vi "Main.vi"() -> ()   [LabVIEW 2019]
doc: "Use this template to build a simple state machine design pattern. Each state executes code and determines which state to transition to."
uses:
  controls/Data.ctl
  controls/State.ctl
  <vilib>/Utility/miscctls.llb/LVPointTypeDef.ctl
panel:
  in  "Prompt Empty":bool
  in  "History":bool
  in  "Advanced":bool
  out "NextEffect3":picture
  out "NextEffect2":picture
  out "NextEffect1":picture
  out "Effect3":picture
  out "Effect2":picture
  out "Effect1":picture
  out "Title":picture
  out "Player Aid":picture
  out "Discard":i32 caption="Discard Deck Size"
  out "Draw":i32 caption="Draw Deck Size"
  out "Value 3":i32
  out "Value 2":i32
  out "Value 1":i32
  in  "Player Reshuffle":bool
  out "Error":errorcluster
  in  "Exit":bool
  in  "Draw Next":bool
  in  "Reset":bool
  out "Scoring3":picture
  out "Scoring2":picture
  out "Scoring1":picture
  out "NumberBack3":picture
  out "NumberBack2":picture
  out "NumberBack1":picture
  out "EffectBack3":picture
  out "EffectBack2":picture
  out "EffectBack1":picture
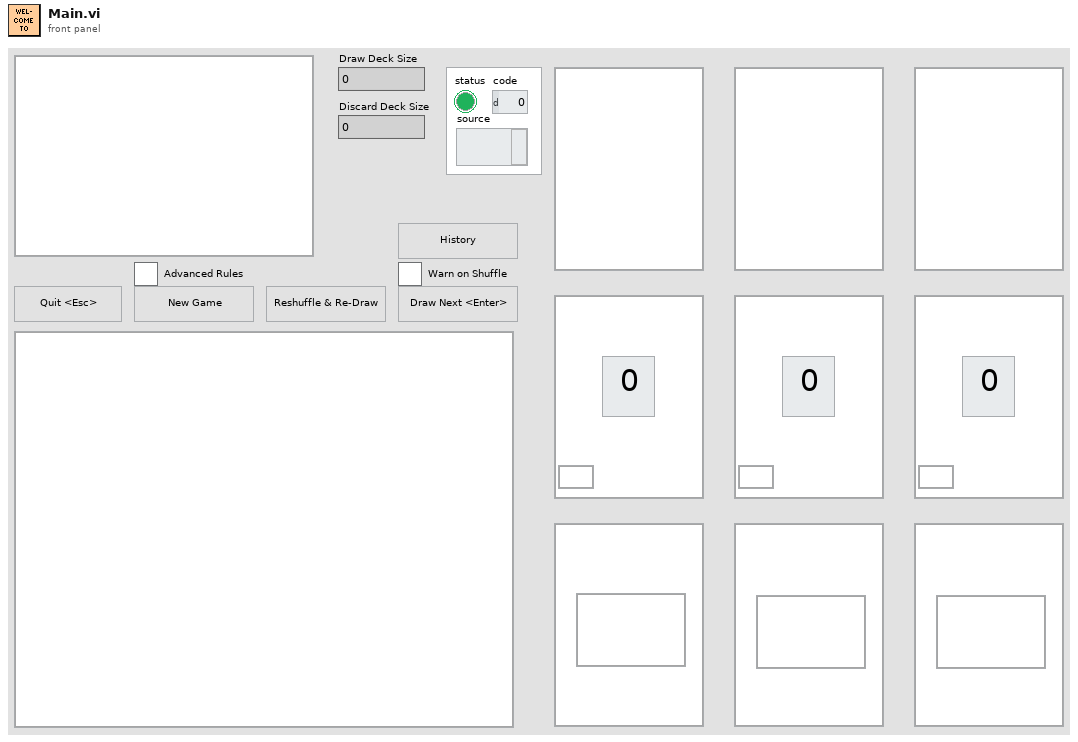
[diagram p1: front panel]
types:
  T1 = typedef "State.ctl" = enum16{"Initialize", "Draw Next Cards", "Shuffle", "Update Display", "Wait for Event", "Reset", "Error", "Exit"}
  T2 = typedef "Data.ctl" = cluster{"Draw Deck":variant[], "Discard Deck":variant[], "Effect Images":variant, "Cards In Draw Deck":i32, "City Card Deck":variant[]}
  T3 = typedef "LVPointTypeDef.ctl" = cluster{"Horizontal":i16, "Vertical":i16}
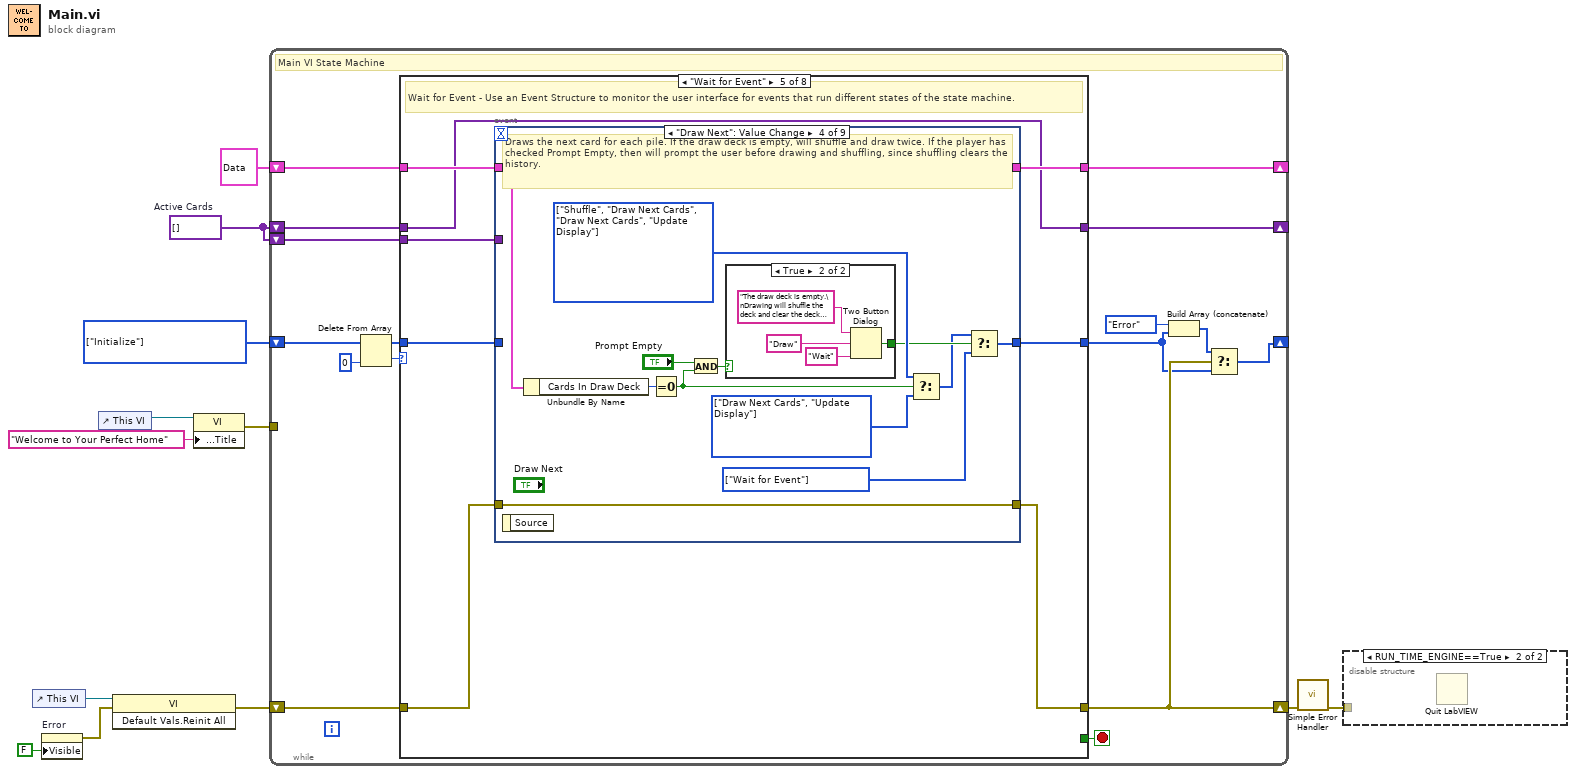
[diagram p0: block diagram]
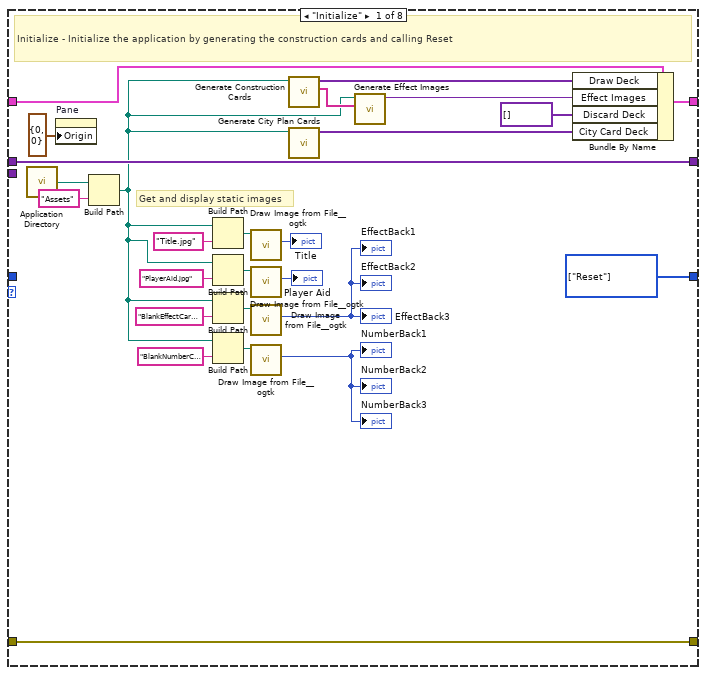
[diagram p3: hidden frame]
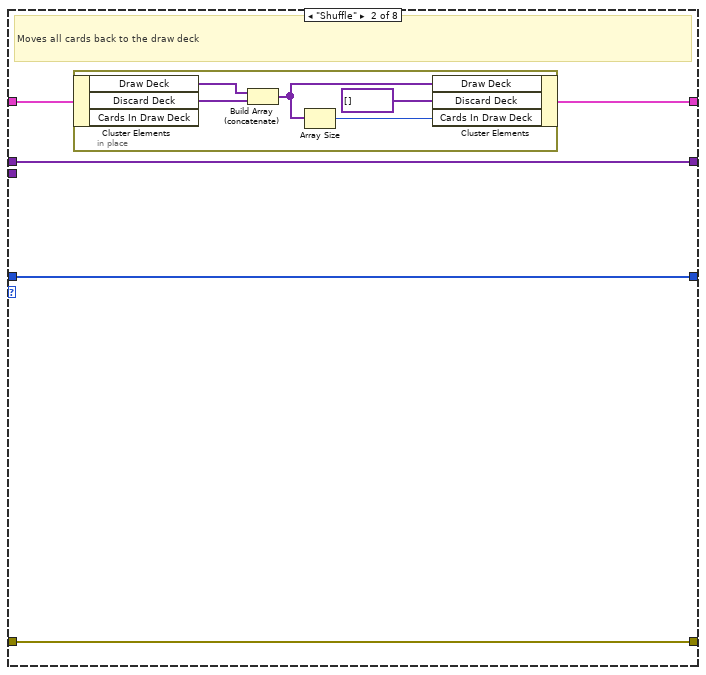
[diagram p4: hidden frame]
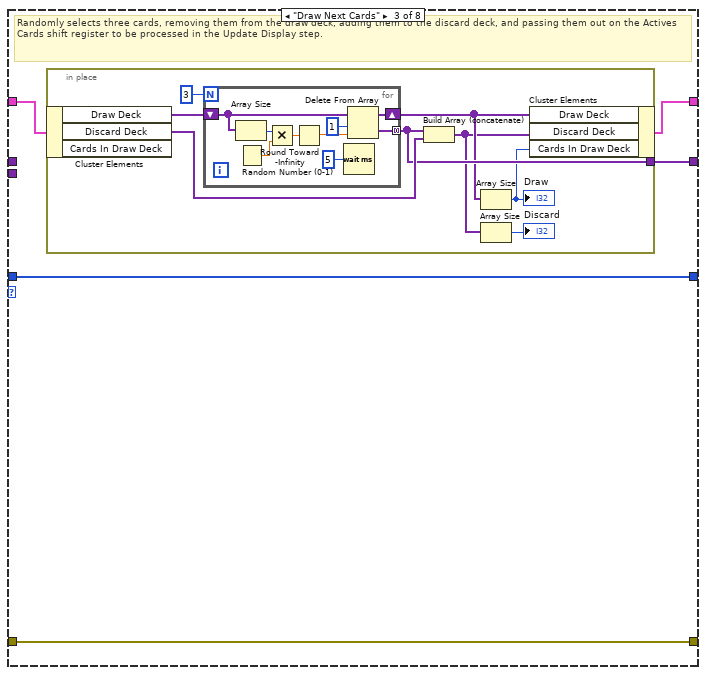
[diagram p5: hidden frame]
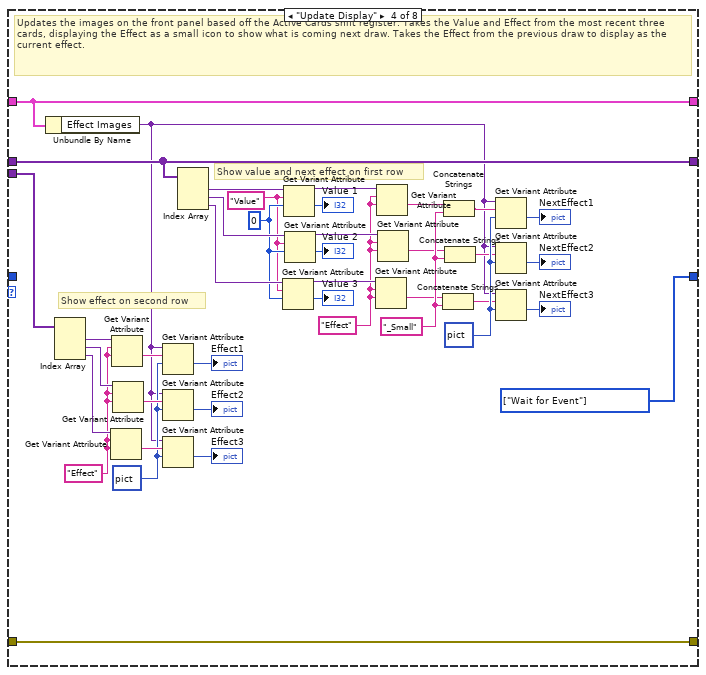
[diagram p6: hidden frame]
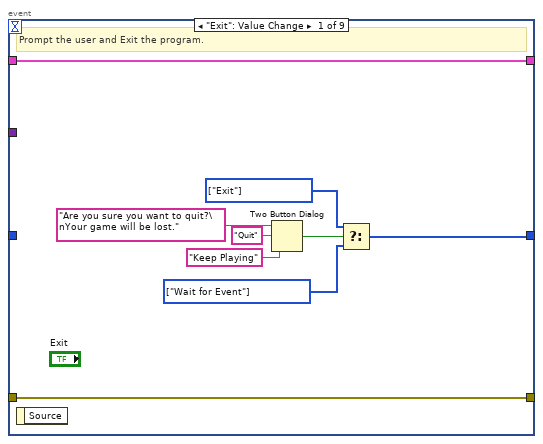
[diagram p7: hidden frame]
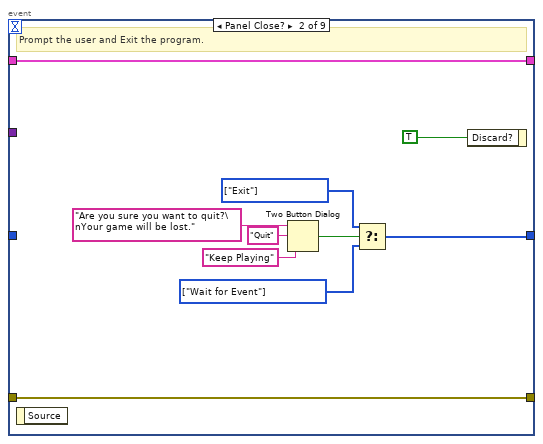
[diagram p8: hidden frame]
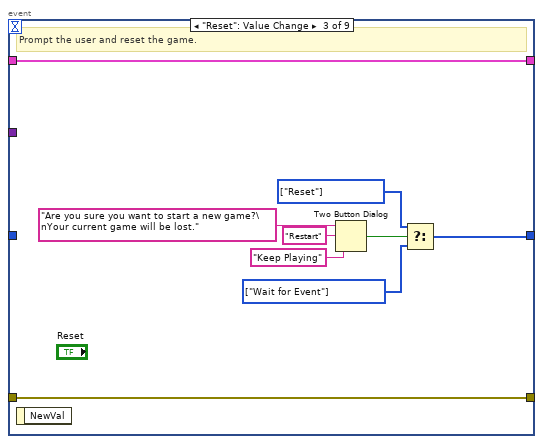
[diagram p9: hidden frame]
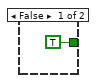
[diagram p10: hidden frame]
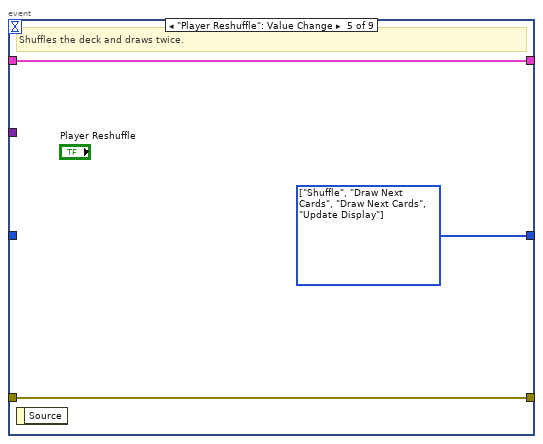
[diagram p11: hidden frame]
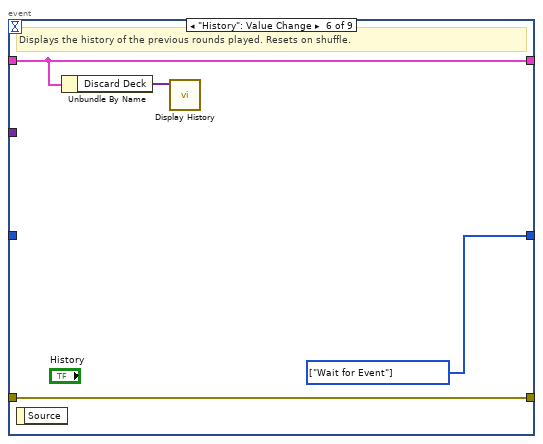
[diagram p12: hidden frame]
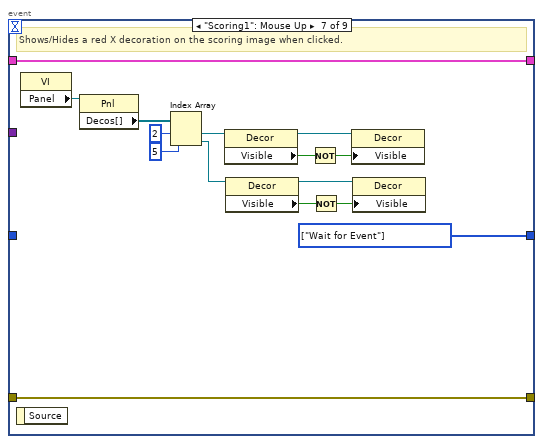
[diagram p13: hidden frame]
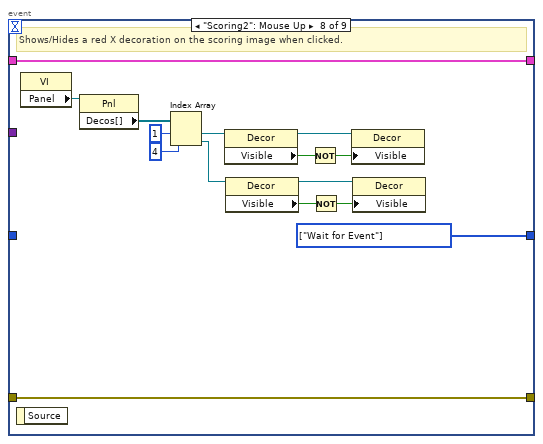
[diagram p14: hidden frame]
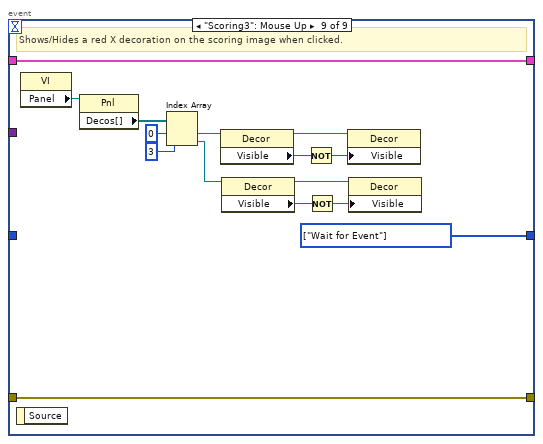
[diagram p15: hidden frame]
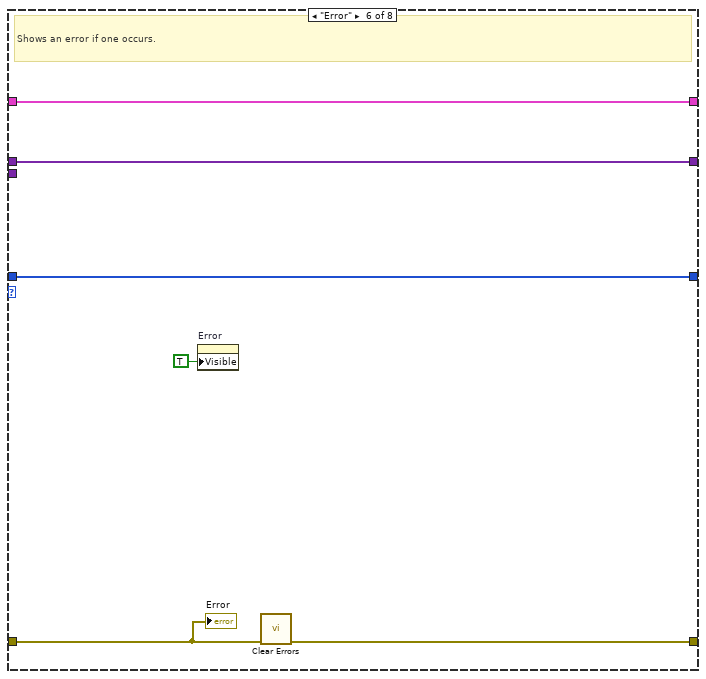
[diagram p16: hidden frame]
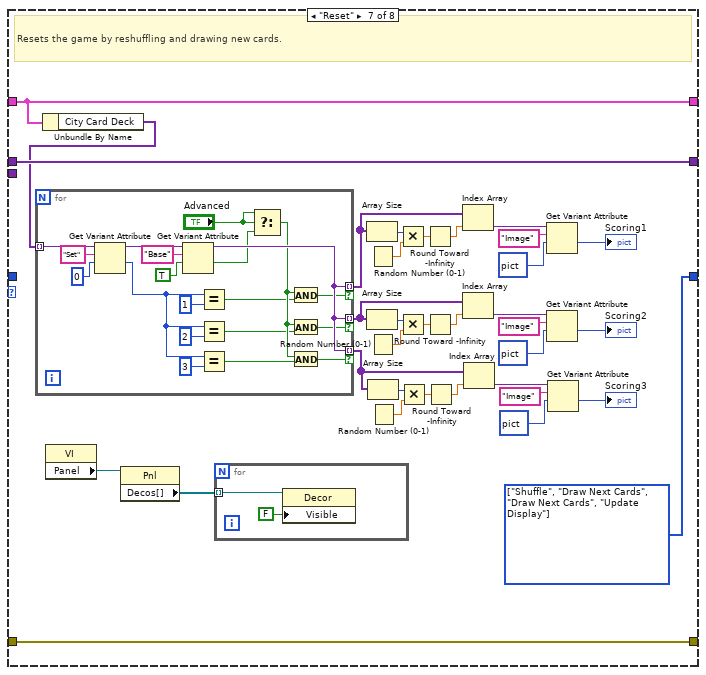
[diagram p17: hidden frame]
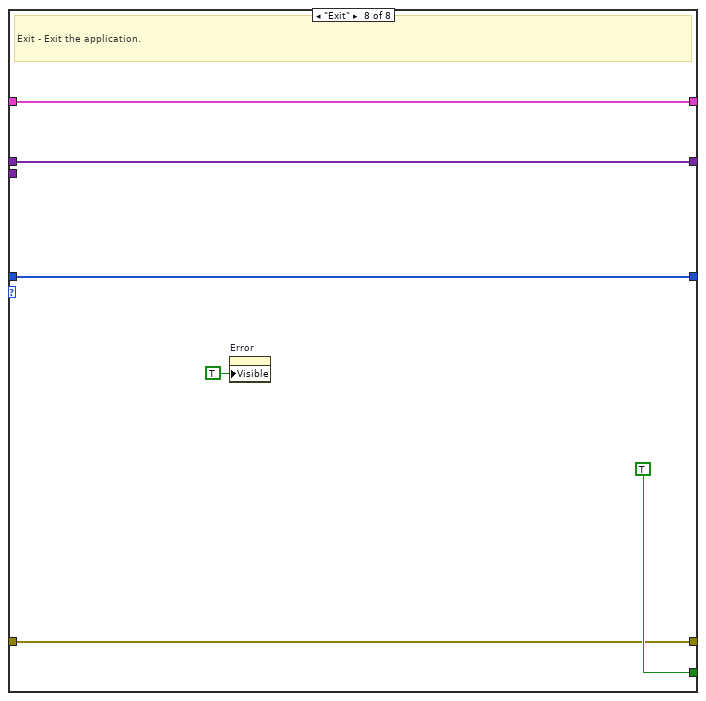
[diagram p18: hidden frame]
diagram:
  w4 = variant[] []  # Active Cards
  w9 = T1[] [enum."Initialize"] items=["Initialize", "Draw Next Cards", "Shuffle", "Update Display", "Wait for Event", "Reset", "Error", "Exit"]
  n1 = control-ref of="This VI"() -> (w8:refnum<vi>)
  n2 = property on="Error" class="Clust (strict)"("Visible"=FALSE) -> (error out=w5:errorcluster)  [unwired: 2 in, 1 out]
  n3 = control-ref of="This VI"() -> (w3:refnum<vi>)
  n4 = invoke class="VI" method="Default Vals.Reinit All"(reference=w8, error in=w5) -> (error out=w7:errorcluster)  [unwired: 1 in, 2 out]
  n5 = property class="VI"(reference=w3, "Front Panel.Title"="Welcome to Your Perfect Home" ("Front Panel Window:Title")) -> (error out=w1:errorcluster)  [unwired: 1 in, 1 out]
  n6 = while {
    shift-right: [w18] -> _
    shift-left: w9 -> [w23]
    shift-right: [w27] -> _
    shift-left: T2 {"Draw Deck"=[], "Discard Deck"=[], "Effect Images"=variant(variant[] []), "Cards In Draw Deck"=0, "City Card Deck"=[]} ("Data") -> [w28]
    shift-right: [w24] -> w11
    shift-left: w7 -> [w26]
    shift-right: [w15] -> _
    shift-left: w4 -> [w14]
    shift-left: w4 -> [w13]
    tunnel: w1 -> [_]
    stop <- w25 stop-if-true
    # "Main VI State Machine"
    n7 = Delete From Array(array=w23, index=0) -> (deleted portion=w21:T1, array with subset deleted=w20:T1[])  [unwired: 1 in]
    n8 = case shown="\"Wait for Event\"" w21 {
      tunnel: [w53 w58 w65 w125 w134 w236 w270 w296] -> w16
      tunnel: [_ _ _ _ _ _ _ TRUE ("Stop Loop")] -> w25
      tunnel: w28 -> [w33 w57 w68 w110 w133 w237 w268 w299]
      tunnel: [w52 w56 w67 w110 w132 w237 w268 w299] -> w27
      tunnel: w26 -> [w54 w59 w69 w126 w131 w234 w271 w297]
      tunnel: [w54 w59 w69 w126 w130 w233 w271 w297] -> w24
      tunnel: w20 -> [_ w58 w65 _ w129 w236 _ w296]
      tunnel: [w51 w55 w66 w121 w128 w232 w269 w294] -> w15
      tunnel: w14 -> [w51 w55 _ w121 w128 w232 w269 w294]
      tunnel: w13 -> [_ _ _ w114 w127 _ _ _]
      frame "Initialize" {
        w53 = T1[] [enum."Reset"] items=["Initialize", "Draw Next Cards", "Shuffle", "Update Display", "Wait for Event", "Reset", "Error", "Exit"] ("Array")
        # "Get and display static images"
        # "Initialize - Initialize the application by generating the construction cards and calling Reset"
        n9 = call <vilib>:"Application Directory.vi"() -> ("Application Directory"=w50:path)
        n10 = property on="Pane" class="Pane"("Origin"=T3 {"Horizontal"=0, "Vertical"=0}) -> ()  [unwired: 2 in, 2 out]
        n11 = Build Path(base path=w50, name or relative path="Assets") -> (appended path=w29:path)
        n12 = Build Path(base path=w29, name or relative path="Title.jpg") -> (appended path=w47:path)
        n13 = Build Path(base path=w29, name or relative path="PlayerAid.jpg") -> (appended path=w45:path)
        n14 = Build Path(base path=w29, name or relative path="BlankEffectCard.jpg") -> (appended path=w40:path)
        n15 = Build Path(base path=w29, name or relative path="BlankNumberCard.jpg") -> (appended path=w39:path)
        n16 = call <userlib>:"Draw Image from File__ogtk.vi"("path to image file"=w47) -> ("new picture"=→"Title":picture)  [unwired: 7 in, 3 out]
        n17 = call <userlib>:"Draw Image from File__ogtk.vi"("path to image file"=w45) -> ("new picture"=→"Player Aid":picture)  [unwired: 7 in, 3 out]
        n18 = call <userlib>:"Draw Image from File__ogtk.vi"("path to image file"=w40) -> ("new picture"=→"EffectBack2" →"EffectBack3" →"EffectBack1":picture)  [unwired: 7 in, 3 out]
        n19 = call <userlib>:"Draw Image from File__ogtk.vi"("path to image file"=w39) -> ("new picture"=→"NumberBack2" →"NumberBack3" →"NumberBack1":picture)  [unwired: 7 in, 3 out]
        n20 = call "Generate Construction Cards.vi"("Path"=w29) -> ("Effect Types"=w35:string[], "Construction Cards"=w32:variant[])  [unwired: 9 in]
        n21 = call "Generate City Plan Cards.vi"("Path"=w29) -> ("City Plan Cards"=w34:variant[])  [unwired: 10 in]
        n22 = call "Generate Effect Images.vi"("Effect Types"=w35, "Path"=w29) -> ("Effect Images"=w31:variant)  [unwired: 9 in]
        n23 = Bundle By Name(cluster=w33, "Draw Deck"=w32, "Effect Images"=w31, "Discard Deck"=variant[] [], "City Card Deck"=w34) -> (w52:T2)
      }
      frame "Shuffle" {
        # "Moves all cards back to the draw deck"
        n24 = in-place {
          n25 = in-place-cluster #1(w57) -> ("Draw Deck"=w62:variant[], "Discard Deck"=w63:variant[])  [unwired: 1 out]
          n26 = Build Array (concatenate)(w62, w63) -> (w60:variant[])
          n27 = Array Size(array=w60) -> (size(s)=w61:i32)
          n28 = in-place-cluster #1("Draw Deck"=w60, "Discard Deck"=variant[] [], "Cards In Draw Deck"=w61) -> (w56:T2)
        }
      }
      frame "Draw Next Cards" {
        # "Randomly selects three cards, removing them from the draw deck, adding them to the discard deck, and passing them out on the Actives Cards shift register to be processed in the Update Display step."
        n29 = in-place {
          in-place-border: [w74] -> w66
          n30 = in-place-cluster #2(w68) -> ("Draw Deck"=w76:variant[], "Discard Deck"=w75:variant[])  [unwired: 1 out]
          n31 = for {
            N: 3 -> [_]
            shift-right: [w80] -> w73
            shift-left: w76 -> [w83]
            tunnel: [w79] -> w74 mode=concatenating
            n32 = Array Size(array=w83) -> (size(s)=w85:i32)
            n33 = Random Number (0-1)() -> (number: 0 to 1=w86:dbl)
            n34 = Multiply(x=w85, y=w86) -> (x*y=w84:dbl)
            n35 = Round Toward -Infinity(1:w84) -> (0:w81:dbl)
            n36 = Wait (ms)(milliseconds to wait=u32 5) -> ()  [unwired: 1 out]
            n37 = Delete From Array(array=w83, length=1, index=w81) -> (deleted portion=w79:variant[], array with subset deleted=w80:variant[])
          }
          n38 = Build Array (concatenate)(w74, w75) -> (w72:variant[])
          n39 = Array Size(array=w73) -> (size(s)=w70:i32)
          "Draw" <- w70
          n40 = Array Size(array=w72) -> (size(s)=→"Discard":i32)
          n41 = in-place-cluster #2("Draw Deck"=w73, "Discard Deck"=w72, "Cards In Draw Deck"=w70) -> (w67:T2)
        }
      }
      frame "Update Display" {
        w94 = picture bytes[61980] ("Effect1")
        w98 = "_Small" ("string")
        w105 = picture bytes[61980] ("Effect1")
        w99 = "Effect" ("name")
        w106 = "Effect" ("name")
        w101 = 0 ("Value 1")
        w100 = "Value" ("name")
        w125 = T1[] [enum."Wait for Event"] items=["Initialize", "Draw Next Cards", "Shuffle", "Update Display", "Wait for Event", "Reset", "Error", "Exit"] ("Array")
        # "Show value and next effect on first row"
        # "Show effect on second row"
        # "Updates the images on the front panel based off the Active Cards shift register. Takes the Value and Effect from the most recent three cards, displaying the Effect as a small icon to show what is coming next draw. Takes the Effect from the previous draw to display as the current effect."
        n42 = Unbundle By Name(w110) -> ("Effect Images"=w90:variant)
        n43 = Index Array(array=w114) -> (element #1=w115:variant, element #2=w116:variant, element #3=w117:variant)  [unwired: 3 in]
        n44 = Get Variant Attribute(Variant=w117, name=w106, default value (empty Variant)=w106) -> (value=w107:string)  [unwired: 1 in, 3 out]
        n45 = Get Variant Attribute(Variant=w115, name=w106, default value (empty Variant)=w106) -> (value=w109:string)  [unwired: 1 in, 3 out]
        n46 = Get Variant Attribute(Variant=w116, name=w106, default value (empty Variant)=w106) -> (value=w108:string)  [unwired: 1 in, 3 out]
        n47 = Get Variant Attribute(Variant=w90, name=w109, default value (empty Variant)=w105) -> (value=→"Effect1":picture)  [unwired: 1 in, 3 out]
        n48 = Get Variant Attribute(Variant=w90, name=w108, default value (empty Variant)=w105) -> (value=→"Effect2":picture)  [unwired: 1 in, 3 out]
        n49 = Get Variant Attribute(Variant=w90, name=w107, default value (empty Variant)=w105) -> (value=→"Effect3":picture)  [unwired: 1 in, 3 out]
        n50 = Index Array(array=w121) -> (element #1=w120:variant, element #2=w119:variant, element #3=w118:variant)  [unwired: 3 in]
        n51 = Get Variant Attribute(Variant=w118, name=w100, default value (empty Variant)=w101) -> (duplicate Variant=w111:variant, value=→"Value 3":i32)  [unwired: 1 in, 2 out]
        n52 = Get Variant Attribute(Variant=w120, name=w100, default value (empty Variant)=w101) -> (duplicate Variant=w113:variant, value=→"Value 1":i32)  [unwired: 1 in, 2 out]
        n53 = Get Variant Attribute(Variant=w119, name=w100, default value (empty Variant)=w101) -> (duplicate Variant=w112:variant, value=→"Value 2":i32)  [unwired: 1 in, 2 out]
        n54 = Get Variant Attribute(Variant=w111, name=w99, default value (empty Variant)=w99) -> (value=w95:string)  [unwired: 1 in, 3 out]
        n55 = Get Variant Attribute(Variant=w113, name=w99, default value (empty Variant)=w99) -> (value=w96:string)  [unwired: 1 in, 3 out]
        n56 = Get Variant Attribute(Variant=w112, name=w99, default value (empty Variant)=w99) -> (value=w97:string)  [unwired: 1 in, 3 out]
        n57 = Concatenate Strings(w95, w98) -> (w91:string)
        n58 = Concatenate Strings(w96, w98) -> (w93:string)
        n59 = Concatenate Strings(w97, w98) -> (w92:string)
        n60 = Get Variant Attribute(Variant=w90, name=w93, default value (empty Variant)=w94) -> (value=→"NextEffect1":picture)  [unwired: 1 in, 3 out]
        n61 = Get Variant Attribute(Variant=w90, name=w92, default value (empty Variant)=w94) -> (value=→"NextEffect2":picture)  [unwired: 1 in, 3 out]
        n62 = Get Variant Attribute(Variant=w90, name=w91, default value (empty Variant)=w94) -> (value=→"NextEffect3":picture)  [unwired: 1 in, 3 out]
      }
      frame "Wait for Event" {
        # "Wait for Event - Use an Event Structure to monitor the user interface for events that run different states of the state machine."
        n63 = event shown="[3] \"Draw Next\": Value Change" {
          selector: _ -> [_ _ _ _ _ _ _ _ _]
          dyn-events: _ -> [_ _ _ _ _ _ _ _ _]
          timeout: _ -> [_ _ _ _ _ _ _ _ _]
          tunnel: [w135 w145 w154 w164 w180 w185 w190 w205 w220] -> w134
          tunnel: w133 -> [w143 w153 w162 w173 w182 w183 w201 w216 w231]
          tunnel: [w143 w153 w162 w173 w182 w183 w201 w216 w231] -> w132
          tunnel: w131 -> [w142 w152 w161 w174 w181 w186 w200 w215 w230]
          tunnel: [w142 w152 w161 w174 w181 w186 w200 w215 w230] -> w130
          tunnel: w129 -> [_ _ _ _ _ _ _ _ _]
          tunnel: w127 -> [_ _ _ _ _ _ _ _ _]
          event "Exit": Value Change {
            w137 = T1[] [enum."Wait for Event"] items=["Initialize", "Draw Next Cards", "Shuffle", "Update Display", "Wait for Event", "Reset", "Error", "Exit"] ("Array")
            w136 = T1[] [enum."Exit"] items=["Initialize", "Draw Next Cards", "Shuffle", "Update Display", "Wait for Event", "Reset", "Error", "Exit"] ("Array")
            # "Prompt the user and Exit the program."
            n64 = event-data() -> ()  [unwired: 1 in, 1 out]
            n65 = Two Button Dialog(message="Are you sure you want to quit?\nYour game will be lost.", 1:"Keep Playing" ("F button name (\"Cancel\")"), 2:"Quit" ("T button name (\"OK\")")) -> (T button?=w138:bool)
            n66 = Select(t=w136, s=w138, f=w137) -> (s? t:f=w135:T1[])
          }
          event Panel Close? {
            w147 = T1[] [enum."Wait for Event"] items=["Initialize", "Draw Next Cards", "Shuffle", "Update Display", "Wait for Event", "Reset", "Error", "Exit"] ("Array")
            w146 = T1[] [enum."Exit"] items=["Initialize", "Draw Next Cards", "Shuffle", "Update Display", "Wait for Event", "Reset", "Error", "Exit"] ("Array")
            # "Prompt the user and Exit the program."
            n67 = event-data() -> ()  [unwired: 1 in, 1 out]
            n68 = Two Button Dialog(message="Are you sure you want to quit?\nYour game will be lost.", 1:"Keep Playing" ("F button name (\"Cancel\")"), 2:"Quit" ("T button name (\"OK\")")) -> (T button?=w148:bool)
            n69 = Select(t=w146, s=w148, f=w147) -> (s? t:f=w145:T1[])
            n70 = event-data("Discard?"=TRUE) -> ()  [unwired: 1 in, 1 out]
          }
          event "Reset": Value Change {
            w156 = T1[] [enum."Wait for Event"] items=["Initialize", "Draw Next Cards", "Shuffle", "Update Display", "Wait for Event", "Reset", "Error", "Exit"] ("Array")
            w155 = T1[] [enum."Reset"] items=["Initialize", "Draw Next Cards", "Shuffle", "Update Display", "Wait for Event", "Reset", "Error", "Exit"] ("Array")
            # "Prompt the user and reset the game."
            n71 = event-data() -> ()  [unwired: 1 in, 1 out]
            n72 = Two Button Dialog(message="Are you sure you want to start a new game?\nYour current game will be lost.", 1:"Keep Playing" ("F button name (\"Cancel\")"), 2:"Restart" ("T button name (\"OK\")")) -> (T button?=w157:bool)
            n73 = Select(t=w155, s=w157, f=w156) -> (s? t:f=w154:T1[])
          }
          event "Draw Next": Value Change {
            w163 = T1[] [enum."Wait for Event"] items=["Initialize", "Draw Next Cards", "Shuffle", "Update Display", "Wait for Event", "Reset", "Error", "Exit"] ("Array")
            w170 = T1[] [enum."Shuffle", enum."Draw Next Cards", enum."Draw Next Cards", enum."Update Display"] items=["Initialize", "Draw Next Cards", "Shuffle", "Update Display", "Wait for Event", "Reset", "Error", "Exit"] ("Array")
            w171 = T1[] [enum."Draw Next Cards", enum."Update Display"] items=["Initialize", "Draw Next Cards", "Shuffle", "Update Display", "Wait for Event", "Reset", "Error", "Exit"] ("Array")
            # "Draws the next card for each pile. If the draw deck is empty, will shuffle and draw twice. If the player has checked Prompt Empty, then will prompt the user before drawing and shuffling, since shuffling clears the history."
            n74 = event-data() -> ()  [unwired: 1 in, 1 out]
            n75 = Unbundle By Name(w173) -> ("Cards In Draw Deck"=w172:i32)
            n76 = Equal To 0?(x=w172) -> (x = 0?=w169:bool)
            n77 = And(x="Prompt Empty", y=w169) -> (x .and. y?=w167:bool)
            n78 = case shown="True" w167 {
              tunnel: [TRUE ("T button?") w176] -> w166
              frame False {
              }
              frame True {
                n79 = Two Button Dialog(message="The draw deck is empty.\nDrawing will shuffle the deck and clear the deck history.", 1:"Wait" ("F button name (\"Cancel\")"), 2:"Draw" ("T button name (\"OK\")")) -> (T button?=w176:bool)
              }
            }
            n80 = Select(t=w170, s=w169, f=w171) -> (s? t:f=w165:T1[])
            n81 = Select(t=w165, s=w166, f=w163) -> (s? t:f=w164:T1[])
          }
          event "Player Reshuffle": Value Change {
            w180 = T1[] [enum."Shuffle", enum."Draw Next Cards", enum."Draw Next Cards", enum."Update Display"] items=["Initialize", "Draw Next Cards", "Shuffle", "Update Display", "Wait for Event", "Reset", "Error", "Exit"] ("Array")
            # "Shuffles the deck and draws twice."
            n82 = event-data() -> ()  [unwired: 1 in, 1 out]
          }
          event "History": Value Change {
            w185 = T1[] [enum."Wait for Event"] items=["Initialize", "Draw Next Cards", "Shuffle", "Update Display", "Wait for Event", "Reset", "Error", "Exit"] ("Array")
            # "Displays the history of the previous rounds played. Resets on shuffle."
            n83 = event-data() -> ()  [unwired: 1 in, 1 out]
            n84 = Unbundle By Name(w183) -> ("Discard Deck"=w184:variant[])
            n85 = call "Display History.vi"("Discard Deck"=w184) -> ()  [unwired: 10 in, 1 out]
          }
          event "Scoring1": Mouse Up {
            w190 = T1[] [enum."Wait for Event"] items=["Initialize", "Draw Next Cards", "Shuffle", "Update Display", "Wait for Event", "Reset", "Error", "Exit"] ("Array")
            # "Shows/Hides a red X decoration on the scoring image when clicked."
            n86 = event-data() -> ()  [unwired: 1 in, 1 out]
            n87 = property class="VI"() -> ("Panel"=w199:refnum<vi>)  [unwired: 2 in, 2 out]
            n88 = property class="Pnl"(reference=w199) -> ("Decos[]"=w198:refnum<vi>[])  [unwired: 1 in, 2 out]
            n89 = Index Array(array=w198, index #1=2 ("index"), index #2=5 ("index")) -> (element #1=w195:refnum<vi>, element #2=w191:refnum<vi>)
            n90 = property class="Decor"(reference=w195) -> (reference out=w192:refnum<vi>, "Visible"=w194:bool)  [unwired: 1 in, 1 out]
            n91 = property class="Decor"(reference=w191) -> (reference out=w189:refnum<vi>, "Visible"=w187:bool)  [unwired: 1 in, 1 out]
            n92 = Not(x=w194) -> (.not. x?=w193:bool)
            n93 = Not(x=w187) -> (.not. x?=w188:bool)
            n94 = property class="Decor"(reference=w192, "Visible"=w193) -> ()  [unwired: 1 in, 2 out]
            n95 = property class="Decor"(reference=w189, "Visible"=w188) -> ()  [unwired: 1 in, 2 out]
          }
          event "Scoring2": Mouse Up {
            w205 = T1[] [enum."Wait for Event"] items=["Initialize", "Draw Next Cards", "Shuffle", "Update Display", "Wait for Event", "Reset", "Error", "Exit"] ("Array")
            # "Shows/Hides a red X decoration on the scoring image when clicked."
            n96 = event-data() -> ()  [unwired: 1 in, 1 out]
            n97 = property class="VI"() -> ("Panel"=w214:refnum<vi>)  [unwired: 2 in, 2 out]
            n98 = property class="Pnl"(reference=w214) -> ("Decos[]"=w213:refnum<vi>[])  [unwired: 1 in, 2 out]
            n99 = Index Array(array=w213, index #1=1 ("index"), index #2=4 ("index")) -> (element #1=w210:refnum<vi>, element #2=w206:refnum<vi>)
            n100 = property class="Decor"(reference=w210) -> (reference out=w207:refnum<vi>, "Visible"=w209:bool)  [unwired: 1 in, 1 out]
            n101 = property class="Decor"(reference=w206) -> (reference out=w204:refnum<vi>, "Visible"=w202:bool)  [unwired: 1 in, 1 out]
            n102 = Not(x=w209) -> (.not. x?=w208:bool)
            n103 = Not(x=w202) -> (.not. x?=w203:bool)
            n104 = property class="Decor"(reference=w207, "Visible"=w208) -> ()  [unwired: 1 in, 2 out]
            n105 = property class="Decor"(reference=w204, "Visible"=w203) -> ()  [unwired: 1 in, 2 out]
          }
          event "Scoring3": Mouse Up {
            w220 = T1[] [enum."Wait for Event"] items=["Initialize", "Draw Next Cards", "Shuffle", "Update Display", "Wait for Event", "Reset", "Error", "Exit"] ("Array")
            # "Shows/Hides a red X decoration on the scoring image when clicked."
            n106 = event-data() -> ()  [unwired: 1 in, 1 out]
            n107 = property class="VI"() -> ("Panel"=w229:refnum<vi>)  [unwired: 2 in, 2 out]
            n108 = property class="Pnl"(reference=w229) -> ("Decos[]"=w228:refnum<vi>[])  [unwired: 1 in, 2 out]
            n109 = Index Array(array=w228, index #1=0 ("index"), index #2=3 ("index")) -> (element #1=w225:refnum<vi>, element #2=w221:refnum<vi>)
            n110 = property class="Decor"(reference=w225) -> (reference out=w222:refnum<vi>, "Visible"=w224:bool)  [unwired: 1 in, 1 out]
            n111 = property class="Decor"(reference=w221) -> (reference out=w219:refnum<vi>, "Visible"=w217:bool)  [unwired: 1 in, 1 out]
            n112 = Not(x=w224) -> (.not. x?=w223:bool)
            n113 = Not(x=w217) -> (.not. x?=w218:bool)
            n114 = property class="Decor"(reference=w222, "Visible"=w223) -> ()  [unwired: 1 in, 2 out]
            n115 = property class="Decor"(reference=w219, "Visible"=w218) -> ()  [unwired: 1 in, 2 out]
          }
        }
      }
      frame "Error" {
        # "Shows an error if one occurs."
        n116 = property on="Error" class="Clust (strict)"("Visible"=TRUE) -> ()  [unwired: 2 in, 2 out]
        n117 = call <vilib>:"Clear Errors.vi"("error in (no error)"=w234) -> ("error out"=w233:errorcluster)  [unwired: 5 in, 1 out]
        "Error" <- w234
      }
      frame "Reset" {
        w270 = T1[] [enum."Shuffle", enum."Draw Next Cards", enum."Draw Next Cards", enum."Update Display"] items=["Initialize", "Draw Next Cards", "Shuffle", "Update Display", "Wait for Event", "Reset", "Error", "Exit"] ("Array")
        # "Resets the game by reshuffling and drawing new cards."
        n118 = Unbundle By Name(w268) -> ("City Card Deck"=w267:variant[])
        n119 = for {
          tunnel: w267 -> [w293] mode=indexing
          tunnel: [w284] -> w266 mode=indexing if=w282
          tunnel: [w284] -> w243 mode=indexing if=w279
          tunnel: [w284] -> w242 mode=indexing if=w278
          n120 = Get Variant Attribute(Variant=w293, name="Set", default value (empty Variant)=0) -> (duplicate Variant=w292:variant, value=w283:i32)  [unwired: 1 in, 2 out]
          n121 = Get Variant Attribute(Variant=w292, name="Base", default value (empty Variant)=TRUE) -> (duplicate Variant=w284:variant, value=w280:bool)  [unwired: 1 in, 2 out]
          n122 = Equal?(x=w283, y=1) -> (x = y?=w276:bool)
          n123 = Equal?(x=w283, y=2) -> (x = y?=w275:bool)
          n124 = Equal?(x=w283, y=3) -> (x = y?=w274:bool)
          n125 = Select(t="Advanced", s="Advanced", f=w280) -> (s? t:f=w277:bool)
          n126 = And(x=w277, y=w276) -> (x .and. y?=w282:bool)
          n127 = And(x=w277, y=w275) -> (x .and. y?=w279:bool)
          n128 = And(x=w277, y=w274) -> (x .and. y?=w278:bool)
        }
        n129 = property class="VI"() -> ("Panel"=w239:refnum<vi>)  [unwired: 2 in, 2 out]
        n130 = property class="Pnl"(reference=w239) -> ("Decos[]"=w238:refnum<vi>[])  [unwired: 1 in, 2 out]
        n131 = for {
          tunnel: w238 -> [w273] mode=indexing
          n132 = property class="Decor"(reference=w273, "Visible"=FALSE) -> ()  [unwired: 1 in, 2 out]
        }
        n133 = Array Size(array=w266) -> (size(s)=w264:i32)
        n134 = Array Size(array=w243) -> (size(s)=w252:i32)
        n135 = Random Number (0-1)() -> (number: 0 to 1=w265:dbl)
        n136 = Random Number (0-1)() -> (number: 0 to 1=w251:dbl)
        n137 = Array Size(array=w242) -> (size(s)=w249:i32)
        n138 = Random Number (0-1)() -> (number: 0 to 1=w250:dbl)
        n139 = Multiply(x=w264, y=w265) -> (x*y=w263:dbl)
        n140 = Multiply(x=w252, y=w251) -> (x*y=w253:dbl)
        n141 = Multiply(x=w249, y=w250) -> (x*y=w248:dbl)
        n142 = Round Toward -Infinity(1:w263) -> (0:w260:dbl)
        n143 = Round Toward -Infinity(1:w253) -> (0:w256:dbl)
        n144 = Round Toward -Infinity(1:w248) -> (0:w245:dbl)
        n145 = Index Array(array=w266, index=w260) -> (element=w262:variant)
        n146 = Index Array(array=w243, index=w256) -> (element=w254:variant)
        n147 = Index Array(array=w242, index=w245) -> (element=w247:variant)
        n148 = Get Variant Attribute(Variant=w262, name="Image", default value (empty Variant)=picture data[5B] ("new picture")) -> (value=→"Scoring1":picture)  [unwired: 1 in, 3 out]
        n149 = Get Variant Attribute(Variant=w254, name="Image", default value (empty Variant)=picture data[5B] ("new picture")) -> (value=→"Scoring2":picture)  [unwired: 1 in, 3 out]
        n150 = Get Variant Attribute(Variant=w247, name="Image", default value (empty Variant)=picture data[5B] ("new picture")) -> (value=→"Scoring3":picture)  [unwired: 1 in, 3 out]
      }
      frame "Exit" {
        # "Exit - Exit the application."
        n151 = property on="Error" class="Clust (strict)"("Visible"=TRUE) -> ()  [unwired: 2 in, 2 out]
      }
    }
    n152 = Build Array (concatenate)(State."Error" ("(Value Not Used)"), w16) -> (w19:T1[])
    n153 = Select(t=w19, s=w24, f=w16) -> (s? t:f=w18:T1[])
  }
  n154 = call <vilib>:"Simple Error Handler.vi"("error in (no error)"=w11) -> ("error out"=w10:errorcluster)  [unwired: 4 in, 4 out]
  n155 = disable-structure shown="RUN_TIME_ENGINE==True" {
    disable-tunnel: w10 -> [_ _]
    frame condition #0 (active) {
    }
    frame condition #1 {
      n156 = Quit LabVIEW() -> ()  [unwired: 1 in]
    }
  }
